vi "ABC Init.vi"(6 "UART":refnum<vi>, 7 "DAQ":tag, 8 "ErrIn":errorcluster, 10 "PortConfig":T1={"BaudRate"=enum."115200", "StopBits"=10, "DataBits"=8, "Parity"=enum."None", "FlowControl"=2, "TimeOut"=1000, "TermChar"=10, "ReadTermEn"=FALSE} {"TermChar" format="%.0x"; "FlowControl" items=["None", "XON/XOFF", "RTS/CTS", "XON/XOFF & RTS/CTS", "DTR/DSR", "XON/XOFF & DTR/DSR"]; "DataBits" min=5 max=8 step=1; "StopBits" items=["1.0"=10, "1.5"=15, "2.0"=20]}, 11 "ComPort":refnum<visa-resource-name>) -> (0 "ErrOut":errorcluster, 3 "DaqTask":refnum<k21>)   [LabVIEW 2020]
uses:
  <userlib>/KQD LabVIEW User/Serial/Controls/SERIAL PortConfig.ctl
  <userlib>/KQD LabVIEW User/Serial/Controls/SERIAL BaudRate.ctl
  <vilib>/DAQmx/create/channels.llb/DAQmx Create Channel (DI-Digital Input).vi
  <userlib>/Amira UART/Amira UART.lvclass
  <userlib>/KQD LabVIEW User/Serial/Serial.lvlib
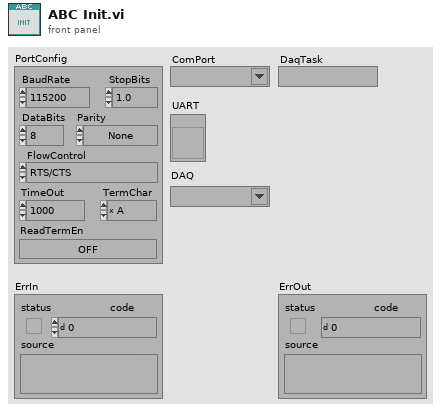
[diagram p1: front panel]
types:
  T1 = typedef "Serial.lvlib/SERIAL PortConfig.ctl" = cluster{"BaudRate":T2, "StopBits":u16, "DataBits":u16, "Parity":enum16{"None", "Odd", "Even", "Mark", "Space"}, "FlowControl":u16, "TimeOut":u32, "TermChar":u8, "ReadTermEn":bool}
  T2 = typedef "SERIAL BaudRate.ctl" = enum16{"2400", "4800", "7200", "9600", "14400", "19200", "28800", "38400", "57600", "115200", "128000", "230400", "460800", "921600"}
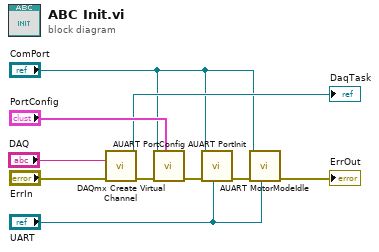
[diagram p0: block diagram]
diagram:
  n1 = call-poly <vilib>:"DAQmx Create Virtual Channel.vi"("lines"="DAQ", "error in"="ErrIn") -> ("task out"=→"DaqTask":refnum<k21>, "error out"=w5:errorcluster)  [unwired: 12 in]
  n2 = call <userlib>:"AUART PortConfig.vi"("Config"="PortConfig", "ErrIn"=w5, "ComPort"="ComPort") -> ("ErrOut"=w10:errorcluster)  [unwired: 8 in]
  n3 = call <userlib>:"AUART PortInit.vi"("UART"="UART", "ErrIn"=w10, "PortIn"="ComPort") -> ("ErrOut"=w9:errorcluster)  [unwired: 7 in, 1 out]
  n4 = call <userlib>:"AUART MotorModeIdle.vi"("UART"="UART", "ErrIn"=w9, "Port"="ComPort") -> ("ErrOut"=→"ErrOut":errorcluster)  [unwired: 7 in, 1 out]
